vi "OEE_SCREEN_2_generate_accumulative_graph_annotations.vi"(10 "Y_annotation_offset":dbl, 11 "graph_values":cluster{dbl[], dbl[]}[](array[cluster])) -> (3 "Array":T1(array[cluster]))   [LabVIEW 2020]
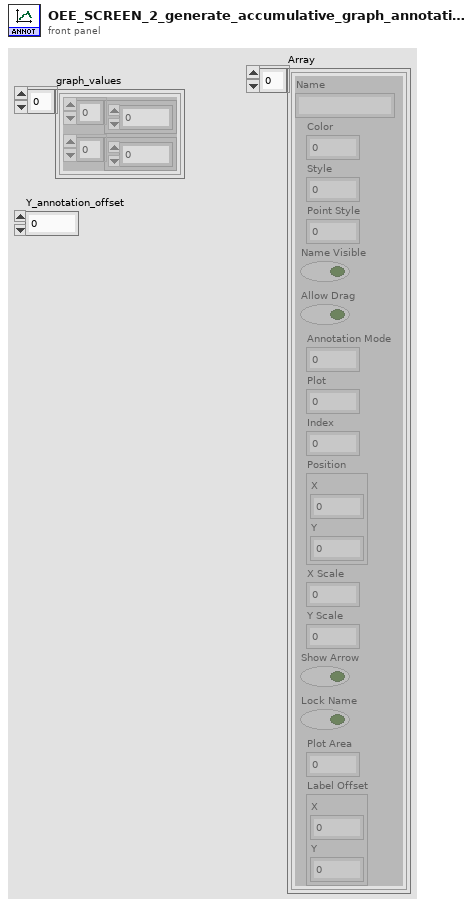
[diagram p1: front panel]
types:
  T1 = cluster{"Name":string, "Color":u32, "Style":u8, "Point Style":u8, "Name Visible":bool, "Allow Drag":bool, "Annotation Mode":u32, "Plot":i32, "Index":i32, "Position":cluster{"X":dbl, "Y":dbl}, "X Scale":u32, "Y Scale":u32, "Show Arrow":bool, "Lock Name":bool, "Plot Area":i32, "Label Offset":cluster{"X":dbl, "Y":dbl}}[]
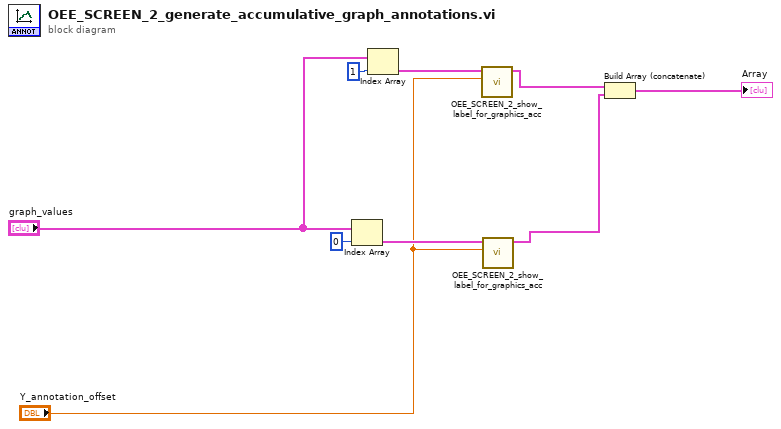
[diagram p0: block diagram]
diagram:
  n1 = Index Array(array="graph_values", index=0) -> (element=w8:cluster{dbl[], dbl[]})
  n2 = Index Array(array="graph_values", index=1) -> (element=w5:cluster{dbl[], dbl[]})
  n3 = call "OEE_SCREEN_2_show_label_for_graphics_acc.vi"("Y_annotation_offset"="Y_annotation_offset", "values"=w5) -> ("Array"=w3:T1)  [unwired: 9 in]
  n4 = call "OEE_SCREEN_2_show_label_for_graphics_acc.vi"("Y_annotation_offset"="Y_annotation_offset", "values"=w8) -> ("Array"=w2:T1)  [unwired: 9 in]
  n5 = Build Array (concatenate)(w3, w2) -> (→"Array":T1)
